vi "Configure Count.vi"(0 "VISA resource name":refnum<visa-resource-name>, 1 "Initial Value Polarity (0: Positive)":i32(ring) items=["Positive", "Negative"], 2 "Samples / Point (1)":i32=1, 5 "Channel (0: chA)":i32(ring) items=["chA", "chB"], 7 "Digital Counter Initial Value (0 FFS)":dbl, 9 "Digital Counter Final Value (0 FFS)":dbl, 11 "error in (no error)":errorcluster, 12 "Enable Negative Final Value (0: Positive)":i32(ring) items=["Positive", "Negative"], 13 "Enable Waveform (T: Enable)":bool=TRUE) -> (4 "VISA resource name out":refnum<visa-resource-name>, 15 "error out":errorcluster)   [LabVIEW 2014, in "Stanford Research SR1.lvlib"]
doc: "Configures the attributes for the Digital Generator Count."
uses:
  Stanford Research SR1.lvlib
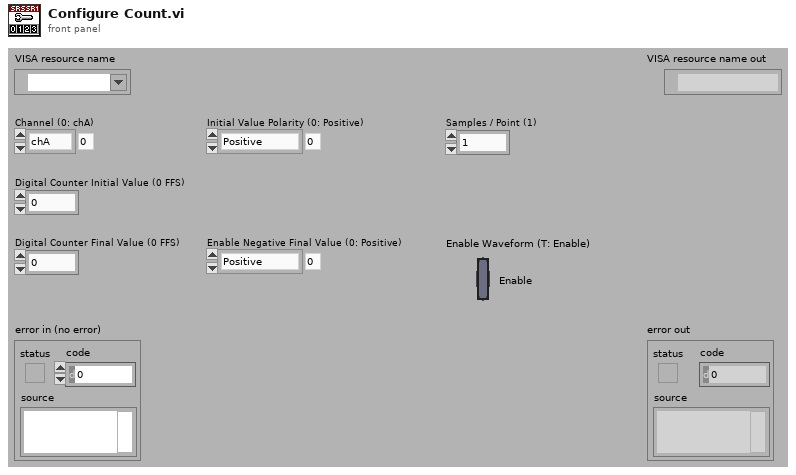
[diagram p1: front panel]
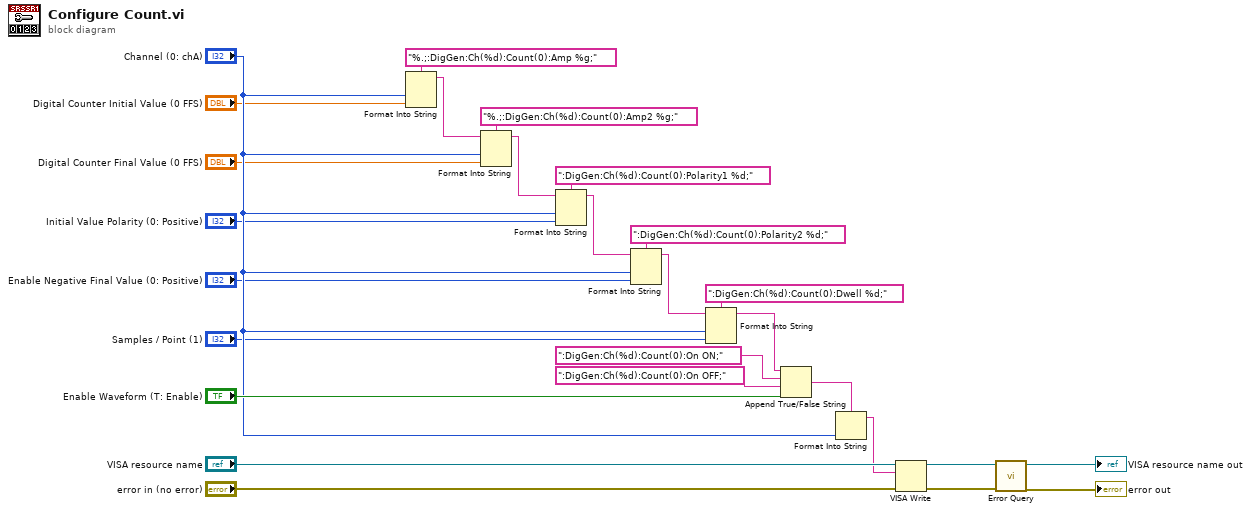
[diagram p0: block diagram]
diagram:
  n1 = Format Into String(format string="%.;:DigGen:Ch(%d):Count(0):Amp %g;", "Channel (0: chA)", "Digital Counter Initial Value (0 FFS)") -> (resulting string=w26:string)  [unwired: 2 in, 1 out]
  n2 = Format Into String(format string="%.;:DigGen:Ch(%d):Count(0):Amp2 %g;", initial string=w26, "Channel (0: chA)", "Digital Counter Final Value (0 FFS)") -> (resulting string=w24:string)  [unwired: 1 in, 1 out]
  n3 = Format Into String(format string=":DigGen:Ch(%d):Count(0):Polarity1 %d;", initial string=w24, "Channel (0: chA)", "Initial Value Polarity (0: Positive)") -> (resulting string=w22:string)  [unwired: 1 in, 1 out]
  n4 = Format Into String(format string=":DigGen:Ch(%d):Count(0):Polarity2 %d;", initial string=w22, "Channel (0: chA)", "Enable Negative Final Value (0: Positive)") -> (resulting string=w20:string)  [unwired: 1 in, 1 out]
  n5 = Format Into String(format string=":DigGen:Ch(%d):Count(0):Dwell %d;", initial string=w20, "Channel (0: chA)", "Samples / Point (1)") -> (resulting string=w18:string)  [unwired: 1 in, 1 out]
  n6 = Append True/False String(1:"Enable Waveform (T: Enable)", 2:":DigGen:Ch(%d):Count(0):On OFF;", 3:":DigGen:Ch(%d):Count(0):On ON;", 4:w18) -> (0:w8:string)
  n7 = Format Into String(format string=w8, "Channel (0: chA)") -> (resulting string=w7:string)  [unwired: 2 in, 1 out]
  n8 = VISA Write(VISA resource name="VISA resource name", write buffer=w7, error in (no error)="error in (no error)") -> (VISA resource name out=w12:refnum<visa-resource-name>, error out=w11:errorcluster)  [unwired: 1 out]
  n9 = call "Error Query.vi"("error in (no error)"=w11, "VISA resource name"=w12) -> ("error out"=→"error out":errorcluster, "VISA resource name out"=→"VISA resource name out":refnum<visa-resource-name>)  [unwired: 6 in, 2 out]
